vi "Server Init Test.vi"() -> (0 "no error":errorcluster, 1 "tags found":bool, 2 "expected execution settings":bool)   [LabVIEW 2013, in "OPC UA Server tests.lvlib"]
doc: "Tests Init override for server configuration"
uses:
  OPC UA Server tests.lvlib
  module/execution/OPC UA Server runtime.lvclass
  <vilib>/OPCUA/server/subVI/supported security policies.ctl
  module/configuration/OPC UA Server configuration.lvclass
  <vilib>/NI/Tag Bus/tag/tag descriptor.lvclass/tag descriptor.ctl
  <vilib>/NI/Tag Bus Module Framework/channel/TBM channel.lvclass/TBM channel.ctl
  <vilib>/NI/Tag Bus/tag/read tag name.vi
  <vilib>/NI/Tag Bus/tag/read data type.vi
  <vilib>/NI/Tag Bus Module Framework/channel/Read channel classification.vi
  <vilib>/NI/Tag Bus/dictionary/data dictionary.lvclass
  <vilib>/NI/Tag Bus Module Framework/channel/TBM channel.lvclass
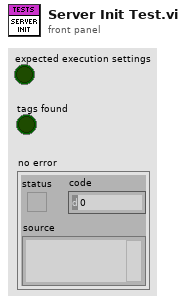
[diagram p1: front panel]
types:
  T1 = typedef "supported security policies.ctl" = cluster{"None":bool, "Sign with Basic128Rsa125":bool, "Sign and Encrypt with Basic128Rsa125":bool, "Sign with Basic256":bool, "Sign and Encrypt with Basic256":bool}
  T2 = cluster{"Client?":bool, "Server Certificates":cluster{"Relative Path?":bool, "Certificate Paths":path[], "Certificate Names":string[]}, "Client Certificates":cluster{"Relative Path?":bool, "Certificate Paths":path[], "Certificate Names":string[]}, "Client Configuration":cluster{"Server Endpoint URL":string, "Security Policy":cluster{"Message Mode":enum16{"None", "Sign", "Sign and Encrypt"}, "Security":enum16{"Basic256", "Basic128Rsa15"}}, "Username/Password":cluster{"Username":string, "Password":string}}, "Server Configuration":cluster{"Server Name":string, "TCP port (49580)":string, "Supported Security Policies":T1}}
  T3 = typedef "TBM channel.lvclass/data tables.ctl" = cluster{"input data":T4, "processing parameter":T4, "processing result":T4, "output data":T4}
  T4 = typedef "tag bus.lvlib/dictionary table pair.ctl" = cluster{"data dictionary":refnum<class "data dictionary.lvclass">, "data table":T5}
  T5 = typedef "tag bus.lvlib/data table.lvlib/data table.ctl" = cluster{"Double":dbl[], "Single":sgl[], "I64":i64[], "I32":i32[], "I16":i16[], "I8":i8[], "U64":u64[], "U32":u32[], "U16":u16[], "U8":u8[], "Boolean":bool[], "String":string[], "Array of Double":cluster{"DBL Array":dbl[]}[], "Array of Single":cluster{"SGL Array":sgl[]}[], "Array of I64":cluster{"I64 Array":i64[]}[], "Array of I32":cluster{"I32 Array":i32[]}[], "Array of I16":cluster{"I16 Array":i16[]}[], "Array of I8":cluster{"I8 Array":i8[]}[], "Array of U64":cluster{"U64 Array":u64[]}[], "Array of U32":cluster{"U32 Array":u32[]}[], "Array of U16":cluster{"U16 Array":u16[]}[], "Array of U8":cluster{"U8 Array":u8[]}[], "Array of Boolean":cluster{"Boolean Array":bool[]}[], "Array of String":cluster{"String Array":string[]}[]}
  T6 = typedef "TBM module execution interface.lvclass/execution settings.ctl" = cluster{"reads inputs":bool, "processes data":bool, "writes outputs":bool}
  T7 = typedef "tag bus.lvlib/tag descriptor.lvclass/Data Type.ctl" = enum16{"Double", "Single", "I64", "I32", "I16", "I8", "U64", "U32", "U16", "U8", "Boolean", "String", "Array of Double", "Array of Single", "Array of I64", "Array of I32", "Array of I16", "Array of I8", "Array of U64", "Array of U32", "Array of U16", "Array of U8", "Array of Boolean", "Array of String"}
  T8 = typedef "TBM channel.lvclass/channel classification.ctl" = enum16{"input data", "output data", "processing parameter", "processing result"}
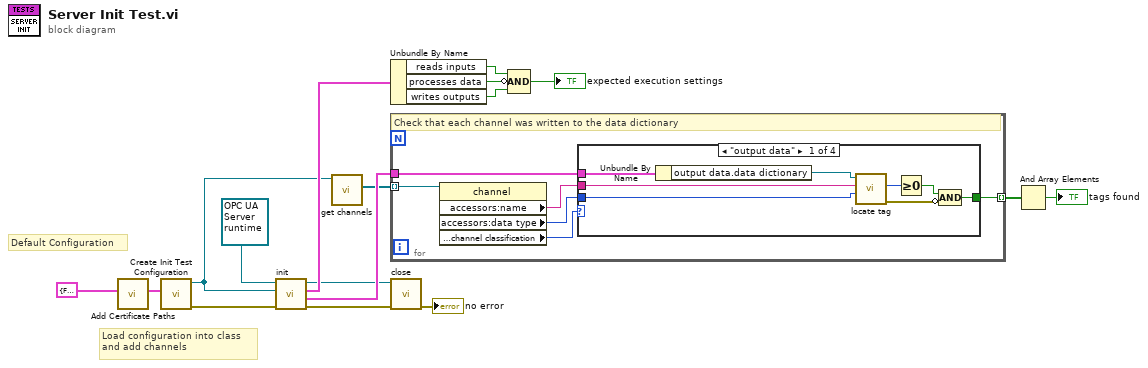
[diagram p0: block diagram]
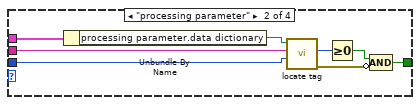
[diagram p2: hidden frame]
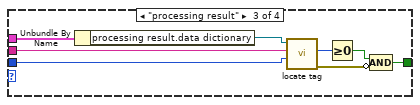
[diagram p3: hidden frame]
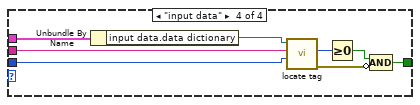
[diagram p4: hidden frame]
diagram:
  # "Load configuration into class\nand add channels"
  # "Default Configuration"
  n1 = call "Add Certificate Paths.vi"("Connection Configuration in"=T2 {"Client?"=FALSE, "Server Certificates"={"Relative Path?"=FALSE, "Certificate Paths"=[path "C:/Users/Administrator/Desktop/OPC-UA-master/OPC-UA-master/Source/testing/Custom OPC UA Tests/Certificates/My Server.der"], "Certificate Names"=[]}, "Client Certificates"={"Relative Path?"=FALSE, "Certificate Paths"=[path "C:/Users/Administrator/Desktop/OPC-UA-master/OPC-UA-master/Source/testing/Custom OPC UA Tests/Certificates/DCAF Client Test Certificate.der"], "Certificate Names"=[]}, "Client Configuration"={"Server Endpoint URL"="", "Security Policy"={"Message Mode"=enum."None", "Security"=enum."Basic256"}, "Username/Password"={"Username"="", "Password"=""}}, "Server Configuration"={"Server Name"="Test", "TCP port (49580)"="49580", "Supported Security Policies"={"None"=TRUE, "Sign with Basic128Rsa125"=FALSE, "Sign and Encrypt with Basic128Rsa125"=FALSE, "Sign with Basic256"=FALSE, "Sign and Encrypt with Basic256"=FALSE}}} ("Connection Configuration")) -> ("Connection Configuration out"=w1:T2)  [unwired: 10 in]
  n2 = call "Create Init Test Configuration.vi"("Connection Configuration"=w1) -> ("error out"=w5:errorcluster, "module"=w4:refnum<class "OPC UA Server configuration.lvclass">)  [unwired: 9 in]
  n3 = call-dynamic "init.vi"("error in"=w5, "TBM module configuration in"=w4, "OPC UA runtime in"=refnum<class "OPC UA Server runtime.lvclass"> refnum ("tag bus configurable plugin module")) -> ("error out"=w9:errorcluster, "data allocations"=w17:T3, "execution settings"=w16:T6, "OPC UA runtime out"=w8:refnum<class "OPC UA Server runtime.lvclass">)  [unwired: 5 in]
  n4 = call-dynamic "get channels.vi"("OPC UA configuration in"=w4) -> ("channels"=w3:refnum<class "TBM channel.lvclass">[])  [unwired: 9 in, 1 out]
  n5 = Unbundle By Name(w16) -> ("reads inputs"=w15:bool, "processes data"=w13:bool, "writes outputs"=w14:bool)
  n6 = for {
    tunnel: w17 -> [w23]
    tunnel: w3 -> [w22] mode=indexing
    tunnel: [w21] -> w11 mode=indexing
    # "Check that each channel was written to the data dictionary"
    n7 = property class="channel"(reference=w22) -> ("accessors:name"=w18:string, "accessors:data type"=w19:T7, "data access:channel classification"=w20:T8)  [unwired: 1 in, 2 out]
    n8 = case shown="\"output data\"" w20 {
      tunnel: w23 -> [w31 w39 w47 w55]
      tunnel: w19 -> [w29 w37 w45 w53]
      tunnel: w18 -> [w28 w36 w44 w52]
      tunnel: [w24 w32 w40 w48] -> w21
      frame "output data" {
        n9 = Unbundle By Name(w31) -> ("output data.data dictionary"=w30:refnum<class "data dictionary.lvclass">)
        n10 = call <vilib>:"locate tag.vi"("data type"=w29, "name"=w28, "data dictionary in"=w30) -> ("error out"=w25:errorcluster, "index"=w27:i32)  [unwired: 6 in, 1 out]
        n11 = Greater Or Equal To 0?(x=w27) -> (x >= 0?=w26:bool)
        n12 = Compound Arithmetic op=AND(w26, invert w25) -> (w24:bool)
      }
      frame "processing parameter" {
        n13 = Unbundle By Name(w39) -> ("processing parameter.data dictionary"=w38:refnum<class "data dictionary.lvclass">)
        n14 = call <vilib>:"locate tag.vi"("data type"=w37, "name"=w36, "data dictionary in"=w38) -> ("error out"=w33:errorcluster, "index"=w35:i32)  [unwired: 6 in, 1 out]
        n15 = Greater Or Equal To 0?(x=w35) -> (x >= 0?=w34:bool)
        n16 = Compound Arithmetic op=AND(w34, invert w33) -> (w32:bool)
      }
      frame "processing result" {
        n17 = Unbundle By Name(w47) -> ("processing result.data dictionary"=w46:refnum<class "data dictionary.lvclass">)
        n18 = call <vilib>:"locate tag.vi"("data type"=w45, "name"=w44, "data dictionary in"=w46) -> ("error out"=w41:errorcluster, "index"=w43:i32)  [unwired: 6 in, 1 out]
        n19 = Greater Or Equal To 0?(x=w43) -> (x >= 0?=w42:bool)
        n20 = Compound Arithmetic op=AND(w42, invert w41) -> (w40:bool)
      }
      frame "input data" {
        n21 = Unbundle By Name(w55) -> ("input data.data dictionary"=w54:refnum<class "data dictionary.lvclass">)
        n22 = call <vilib>:"locate tag.vi"("data type"=w53, "name"=w52, "data dictionary in"=w54) -> ("error out"=w49:errorcluster, "index"=w51:i32)  [unwired: 6 in, 1 out]
        n23 = Greater Or Equal To 0?(x=w51) -> (x >= 0?=w50:bool)
        n24 = Compound Arithmetic op=AND(w50, invert w49) -> (w48:bool)
      }
    }
  }
  n25 = call-dynamic "close.vi"("error in"=w9, "OPC UA runtime in"=w8) -> ("error out"=→"no error":errorcluster)  [unwired: 9 in]
  n26 = Compound Arithmetic op=AND(w15, invert w13, w14) -> (→"expected execution settings":bool)
  n27 = And Array Elements(Boolean array=w11) -> (logical AND=→"tags found":bool)
